vi "Config Parse.vi"(0 "Config File Path":path=path "C:/Automation/Configurations/Cenaturo.config", 11 "Error In":errorcluster) -> (4 "Pass/Fail?":bool, 6 "Report Text":string, 8 "Centauro_config":T1, 15 "Error Out":errorcluster)   [LabVIEW 2016, in "Centauro.lvlib"]
uses:
  Projects/Centauro.lvlib
  type defs/Config.ctl
  <vilib>/Utility/config.llb/Read Key (String).vi
  <vilib>/Utility/config.llb/Read Key (Boolean).vi
  <vilib>/Utility/config.llb/NI_LVConfig.lvlib
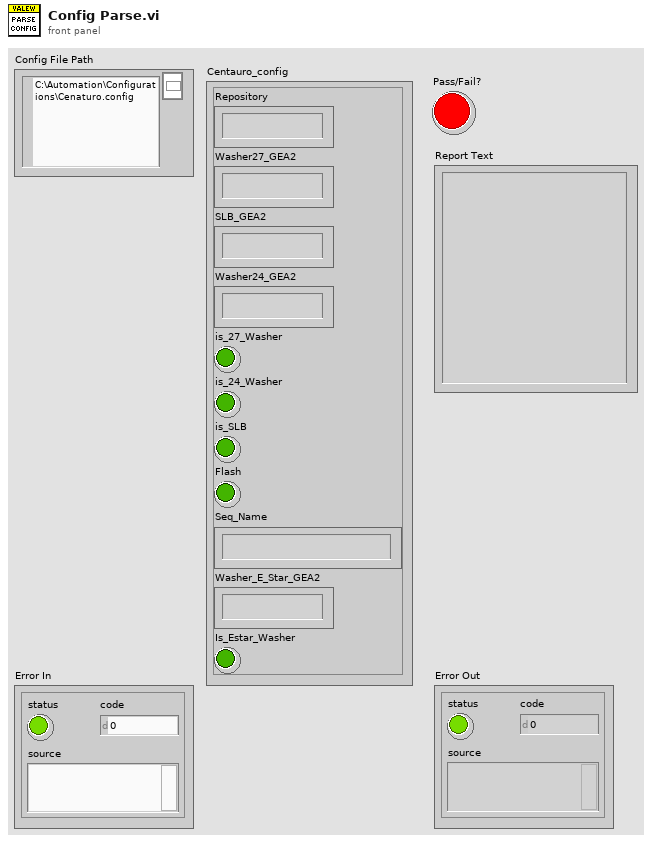
[diagram p1: front panel]
types:
  T1 = typedef "Centauro.lvlib/Config.ctl" = cluster{"Repository":string, "Washer27_GEA2":string, "SLB_GEA2":string, "Washer24_GEA2":string, "is_27_Washer":bool, "is_24_Washer":bool, "is_SLB":bool, "Flash":bool, "Seq_Name":string, "Washer_E_Star_GEA2":string, "Is_Estar_Washer":bool}
  T2 = typedef "NI_LVConfig.lvlib/Config Data RefNum.ctl" = refnum<k1>
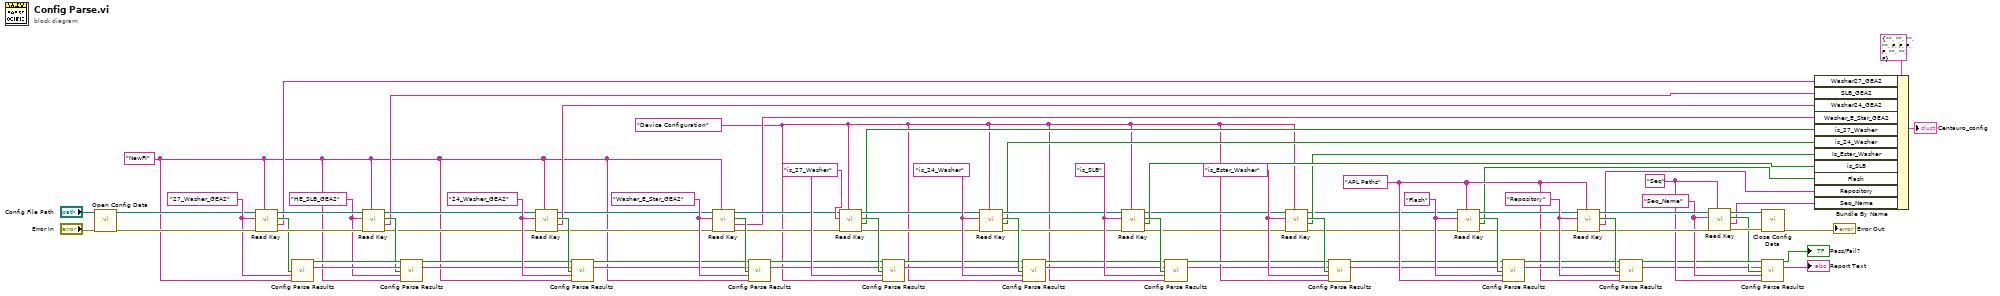
[diagram p0: block diagram]
diagram:
  w11 = "is_Estar_Washer" ("key")
  w22 = "Washer_E_Star_GEA2" ("key")
  w42 = "Seq_Name" ("key")
  w41 = "Seq" ("section")
  w53 = "Repository" ("key")
  w63 = "is_SLB" ("key")
  w66 = "is_24_Washer" ("key")
  w71 = "24_Washer_GEA2" ("key")
  w73 = "Flash" ("key")
  w38 = "APL Paths" ("section")
  w75 = "is_27_Washer" ("key")
  w5 = "Device Configuration" ("section")
  w77 = "HE_SLB_GEA2" ("key")
  w82 = "27_Washer_GEA2" ("key")
  w14 = "NewFI" ("section")
  n1 = call <vilib>:"Open Config Data.vi"("error in (no error)"="Error In", "configuration file path"="Config File Path") -> ("error out"=w85:errorcluster, "refnum"=w47:T2)  [unwired: 7 in, 1 out]
  n2 = call-poly <vilib>:"Read Key.vi"("section"=w14, "error in (no error)"=w85, "key"=w82, "refnum"=w47) -> ("error out"=w86:errorcluster, "value"=w29:string, "found?"=w81:bool, "refnum out"=w87:T2)  [unwired: 4 in]
  n3 = call "Config Parse Results.vi"("found?"=w81, "key"=w82, "section"=w14) -> ("Pass/Fail"=w80:bool, "Report Text"=w79:string)  [unwired: 11 in]
  n4 = call-poly <vilib>:"Read Key.vi"("section"=w14, "error in (no error)"=w86, "key"=w77, "refnum"=w87) -> ("error out"=w69:errorcluster, "value"=w28:string, "found?"=w78:bool, "refnum out"=w70:T2)  [unwired: 4 in]
  n5 = call "Config Parse Results.vi"("Previous Pass/Fail"=w80, "Previous Report Text"=w79, "found?"=w78, "key"=w77, "section"=w14) -> ("Pass/Fail"=w68:bool, "Report Text"=w67:string)  [unwired: 9 in]
  n6 = call-poly <vilib>:"Read Key.vi"("section"=w14, "error in (no error)"=w69, "key"=w71, "refnum"=w70) -> ("error out"=w21:errorcluster, "value"=w27:string, "found?"=w72:bool, "refnum out"=w20:T2)  [unwired: 4 in]
  n7 = call "Config Parse Results.vi"("Previous Pass/Fail"=w68, "Previous Report Text"=w67, "found?"=w72, "key"=w71, "section"=w14) -> ("Pass/Fail"=w16:bool, "Report Text"=w18:string)  [unwired: 9 in]
  n8 = call-poly <vilib>:"Read Key.vi"("section"=w14, "error in (no error)"=w21, "key"=w22, "refnum"=w20) -> ("value"=w13:string, "found?"=w23:bool, "refnum out"=w19:T2)  [unwired: 4 in, 1 out]
  n9 = call "Config Parse Results.vi"("Previous Pass/Fail"=w16, "Previous Report Text"=w18, "found?"=w23, "key"=w22, "section"=w14) -> ("Pass/Fail"=w15:bool, "Report Text"=w17:string)  [unwired: 9 in]
  n10 = call-poly <vilib>:"Read Key.vi"("section"=w5, "error in (no error)"=w21, "key"=w75, "refnum"=w19) -> ("error out"=w60:errorcluster, "value"=w34:bool, "found?"=w76:bool, "refnum out"=w62:T2)  [unwired: 4 in]
  n11 = call "Config Parse Results.vi"("Previous Pass/Fail"=w15, "Previous Report Text"=w17, "found?"=w76, "key"=w75, "section"=w5) -> ("Pass/Fail"=w58:bool, "Report Text"=w57:string)  [unwired: 9 in]
  n12 = call-poly <vilib>:"Read Key.vi"("section"=w5, "error in (no error)"=w60, "key"=w66, "refnum"=w62) -> ("error out"=w59:errorcluster, "value"=w33:bool, "found?"=w65:bool, "refnum out"=w61:T2)  [unwired: 4 in]
  n13 = call "Config Parse Results.vi"("Previous Pass/Fail"=w58, "Previous Report Text"=w57, "found?"=w65, "key"=w66, "section"=w5) -> ("Pass/Fail"=w56:bool, "Report Text"=w55:string)  [unwired: 9 in]
  n14 = call-poly <vilib>:"Read Key.vi"("section"=w5, "error in (no error)"=w59, "key"=w63, "refnum"=w61) -> ("error out"=w2:errorcluster, "value"=w24:bool, "found?"=w64:bool, "refnum out"=w9:T2)  [unwired: 4 in]
  n15 = call "Config Parse Results.vi"("Previous Pass/Fail"=w56, "Previous Report Text"=w55, "found?"=w64, "key"=w63, "section"=w5) -> ("Pass/Fail"=w7:bool, "Report Text"=w4:string)  [unwired: 9 in]
  n16 = call-poly <vilib>:"Read Key.vi"("section"=w5, "error in (no error)"=w2, "key"=w11, "refnum"=w9) -> ("error out"=w1:errorcluster, "value"=w10:bool, "found?"=w12:bool, "refnum out"=w8:T2)  [unwired: 4 in]
  n17 = call "Config Parse Results.vi"("Previous Pass/Fail"=w7, "Previous Report Text"=w4, "found?"=w12, "key"=w11, "section"=w5) -> ("Pass/Fail"=w6:bool, "Report Text"=w3:string)  [unwired: 9 in]
  n18 = call-poly <vilib>:"Read Key.vi"("section"=w38, "error in (no error)"=w1, "key"=w73, "refnum"=w8) -> ("error out"=w48:errorcluster, "value"=w25:bool, "found?"=w74:bool, "refnum out"=w49:T2)  [unwired: 4 in]
  n19 = call "Config Parse Results.vi"("Previous Pass/Fail"=w6, "Previous Report Text"=w3, "found?"=w74, "key"=w73, "section"=w38) -> ("Pass/Fail"=w51:bool, "Report Text"=w50:string)  [unwired: 9 in]
  n20 = call-poly <vilib>:"Read Key.vi"("section"=w38, "error in (no error)"=w48, "key"=w53, "refnum"=w49) -> ("error out"=w46:errorcluster, "value"=w26:string, "found?"=w54:bool, "refnum out"=w44:T2)  [unwired: 4 in]
  n21 = call "Config Parse Results.vi"("Previous Pass/Fail"=w51, "Previous Report Text"=w50, "found?"=w54, "key"=w53, "section"=w38) -> ("Pass/Fail"=w40:bool, "Report Text"=w35:string)  [unwired: 9 in]
  n22 = call-poly <vilib>:"Read Key.vi"("section"=w41, "error in (no error)"=w46, "key"=w42, "refnum"=w44) -> ("error out"=w45:errorcluster, "value"=w30:string, "found?"=w39:bool, "refnum out"=w43:T2)  [unwired: 4 in]
  n23 = call "Config Parse Results.vi"("Previous Pass/Fail"=w40, "Previous Report Text"=w35, "found?"=w39, "key"=w42, "section"=w41) -> ("Pass/Fail"=→"Pass/Fail?":bool, "Report Text"=→"Report Text":string)  [unwired: 9 in]
  n24 = call <vilib>:"Close Config Data.vi"("error in (no error)"=w45, "refnum"=w43) -> ("error out"=→"Error Out":errorcluster)  [unwired: 8 in, 1 out]
  n25 = Bundle By Name(cluster=T1 {"Repository"="", "Washer27_GEA2"="", "SLB_GEA2"="", "Washer24_GEA2"="", "is_27_Washer"=FALSE, "is_24_Washer"=FALSE, "is_SLB"=FALSE, "Flash"=FALSE, "Seq_Name"="", "Washer_E_Star_GEA2"="", "Is_Estar_Washer"=FALSE} ("VALEW_config"), "Washer27_GEA2"=w29, "SLB_GEA2"=w28, "Washer24_GEA2"=w27, "Washer_E_Star_GEA2"=w13, "is_27_Washer"=w34, "is_24_Washer"=w33, "Is_Estar_Washer"=w10, "is_SLB"=w24, "Flash"=w25, "Repository"=w26, "Seq_Name"=w30) -> (→"Centauro_config":T1)
